vi "Set Window Position.vi"(8 "error in":errorcluster, 11 "VI Reference":refnum<vi>) -> (0 "error out":errorcluster)   [LabVIEW 2020, in "Peek Window.lvlib"]
uses:
  Peek Window.lvlib
  <resource>/dialog/lvconfig.llb/LV Config Read String.vi
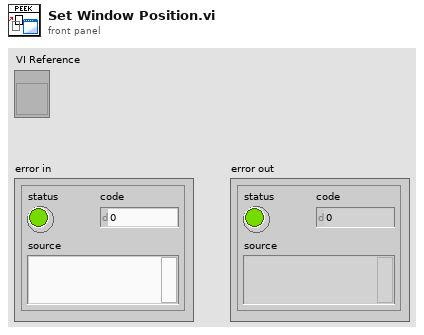
[diagram p1: front panel]
types:
  T1 = cluster{"Left":i16, "Top":i16, "Right":i16, "Bottom":i16}
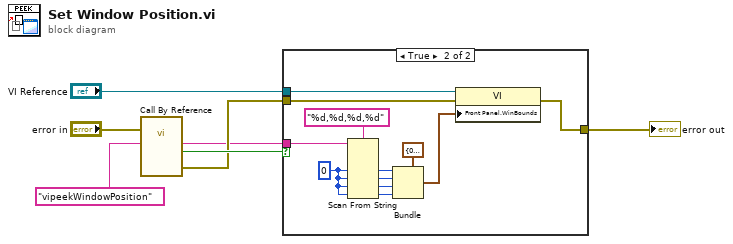
[diagram p0: block diagram]
diagram:
  n1 = call-by-ref "?"(error in="error in", "key"="vipeekWindowPosition" ("Name")) -> ("error out"=w2:errorcluster, "found?"=w3:bool, "value"=w1:string)  [unwired: 5 in, 2 out]
  n2 = case shown="True" w3 {
    tunnel: "VI Reference" -> [_ w20]
    tunnel: [w8 w19] -> w6
    tunnel: w2 -> [w8 w18]
    tunnel: w1 -> [_ w10]
    frame False {
    }
    frame True {
      w16 = i16 0 ("default value 1")
      n3 = Scan From String(format string="%d,%d,%d,%d", input string=w10, default 1=w16, default 2=w16, default 3=w16, default 4=w16) -> (output 1=w15:i16, output 2=w14:i16, output 3=w13:i16, output 4=w12:i16)  [unwired: 2 in, 3 out]
      n4 = Bundle(cluster=T1 {"Left"=0, "Top"=0, "Right"=0, "Bottom"=0} ("Front Panel.PanelBounds"), "Left"=w15, "Top"=w14, "Right"=w13, "Bottom"=w12) -> (w9:T1)
      n5 = property class="VI"(reference=w20, error in=w18, "Front Panel.WinBounds"=w9) -> (error out=w19:errorcluster)  [unwired: 1 out]
    }
  }
  "error out" <- w6
